vi "Config Commutate.vi"(8 "error in":errorcluster, 10 "Commutate (Line Reject)":i32(ring) items=["Off", "Line Reject", "Asynchrounous"], 11 "VISA resource name":refnum<visa-resource-name>) -> (0 "error out":errorcluster, 3 "VISA resource name out":refnum<visa-resource-name>)   [LabVIEW 2017, in "Andeen-Hagerling 2700.lvlib"]
doc: "This VI sets the commutate feature of the bridge. The commutate feature periodically reverses the applied bridge signal. This makes the bridge signal distinguishable from external interference near either the line or bridge frequency. The bridge then rejects the interference."
uses:
  Andeen-Hagerling 2700.lvlib
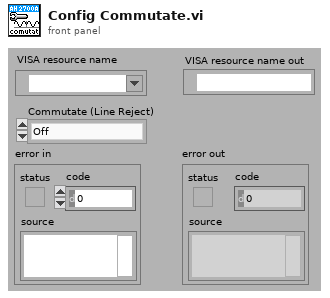
[diagram p1: front panel]
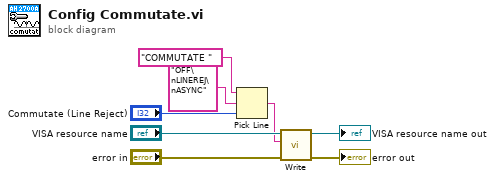
[diagram p0: block diagram]
diagram:
  n1 = Pick Line(string ("")="COMMUTATE ", multi-line string="OFF\nLINEREJ\nASYNC", line index="Commutate (Line Reject)") -> (output string=w3:string)
  n2 = call "Write.vi"("error in"="error in", "command"=w3, "VISA resource name"="VISA resource name") -> ("error out"=→"error out":errorcluster, "VISA resource name out"=→"VISA resource name out":refnum<visa-resource-name>)  [unwired: 7 in]
